vi "Convert_DateTime.vi"(8 "error in (no error)":errorcluster, 11 "Date in (DD/MM/YYYY hh:mm:ss)":string) -> (0 "error out":errorcluster, 3 "Date OUT (YYYY:MM:DD hh:mm:ss)":string)   [LabVIEW 2025]
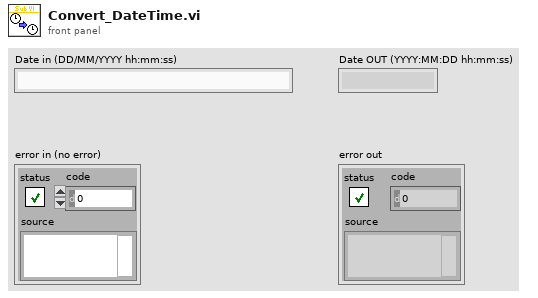
[diagram p1: front panel]
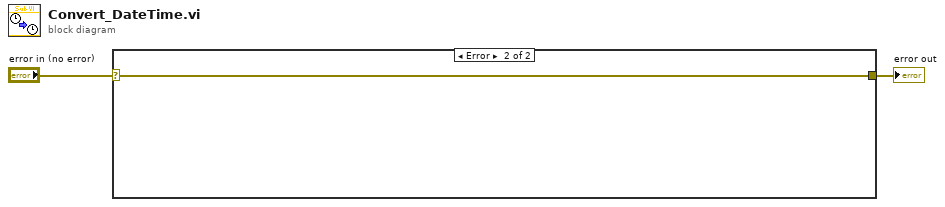
[diagram p0: block diagram]
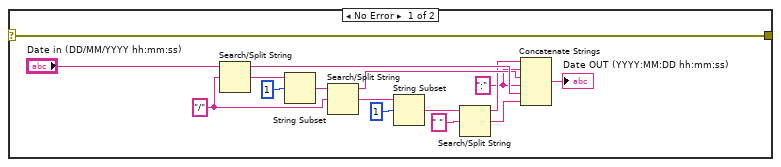
[diagram p2: hidden frame]
diagram:
  n1 = case shown="Error" "error in (no error)" {
    selector: "error in (no error)" -> [w3 w19]
    tunnel: [w3 w19] -> w2
    frame No Error {
      w8 = ":" ("string")
      w4 = "/" ("search string/char (-)")
      n2 = Search/Split String(string="Date in (DD/MM/YYYY hh:mm:ss)", search string/char (-)=w4) -> (substring before match=w16:string, match + rest of string=w10:string)  [unwired: 1 in, 1 out]
      n3 = String Subset(string=w10, offset (0)=1) -> (substring=w11:string)  [unwired: 1 in]
      n4 = Search/Split String(string=w11, search string/char (-)=w4) -> (substring before match=w15:string, match + rest of string=w12:string)  [unwired: 1 in, 1 out]
      n5 = String Subset(string=w12, offset (0)=1) -> (substring=w13:string)  [unwired: 1 in]
      n6 = Search/Split String(string=w13, search string/char (-)=" ") -> (substring before match=w14:string, match + rest of string=w17:string)  [unwired: 1 in, 1 out]
      n7 = Concatenate Strings(w14, w8, w15, w8, w16, w17) -> (→"Date OUT (YYYY:MM:DD hh:mm:ss)":string)
    }
    frame Error {
    }
  }
  "error out" <- w2
